vi "Read Indicator.vi"(5 "High Address":u32 format="%08x", 7 "Base Address":u32 format="%08x", 11 "Address":u32 format="%08x") -> (0 "Error":bool, 3 "Data":i32 format="%08x")   [LabVIEW 2011]
uses:
  Globals.vi
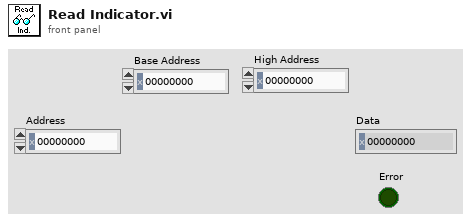
[diagram p1: front panel]
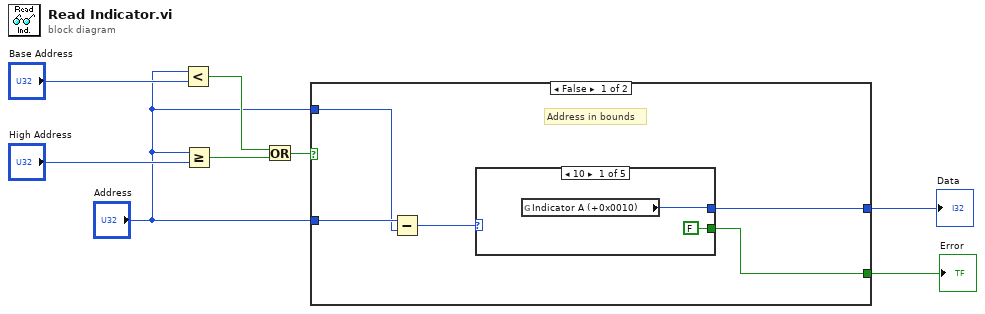
[diagram p0: block diagram]
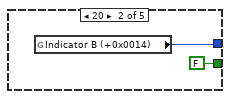
[diagram p2: hidden frame]
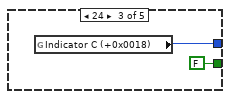
[diagram p3: hidden frame]
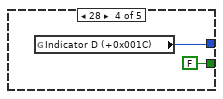
[diagram p4: hidden frame]
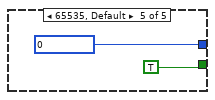
[diagram p5: hidden frame]
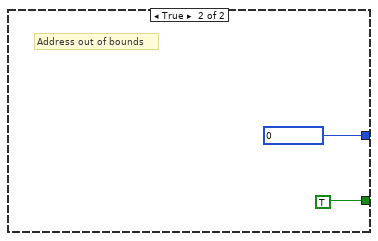
[diagram p6: hidden frame]
diagram:
  n1 = Less?(x="Address", y="Base Address") -> (x < y?=w6:bool)
  n2 = Greater Or Equal?(x="Address", y="High Address") -> (x >= y?=w7:bool)
  n3 = Or(x=w6, y=w7) -> (x .or. y?=w8:bool)
  n4 = case shown="False" w8 {
    tunnel: [w9 TRUE ("Error")] -> w3
    tunnel: "Address" -> [w13 _]
    tunnel: "Address" -> [w12 _]
    tunnel: [w10 0 ("Data")] -> w1
    frame False {
      # "Address in bounds"
      n5 = Subtract(x=w13, y=w12) -> (x-y=w11:u32)
      n6 = case shown="10" w11 {
        tunnel: [w15 w17 w19 w21 0 ("Data")] -> w10
        tunnel: [FALSE ("Error") FALSE ("Error") FALSE ("Error") FALSE ("Error") TRUE ("Error")] -> w9
        frame 16 {
          n7 = global read "Globals.vi" "Indicator A (+0x0010)"() -> (w15:u32)
        }
        frame 20 {
          n8 = global read "Globals.vi" "Indicator B (+0x0014)"() -> (w17:u32)
        }
        frame 24 {
          n9 = global read "Globals.vi" "Indicator C (+0x0018)"() -> (w19:u32)
        }
        frame 28 {
          n10 = global read "Globals.vi" "Indicator D (+0x001C)"() -> (w21:u32)
        }
        frame 65535, Default {
        }
      }
    }
    frame True {
      # "Address out of bounds"
    }
  }
  "Data" <- w1
  "Error" <- w3
